vi "Create.vi"(7 "Registry Name":string, 8 "error in (no error)":errorcluster) -> (0 "error out":errorcluster, 3 "Process Collector out":refnum<class "Process Collector.lvclass">)   [LabVIEW 2020, in "Collector.lvlib" / "Process Collector.lvclass"]
uses:
  Process Collector.lvclass
  C:/Github-locals/PromVIEW/src/collector/collectable/Collectable.lvclass
  Process Collector.lvclass/Process Collector.ctl
  <vilib>/regexp/Match Regular Expression.xnode
  registry/session/Registry Session.lvclass
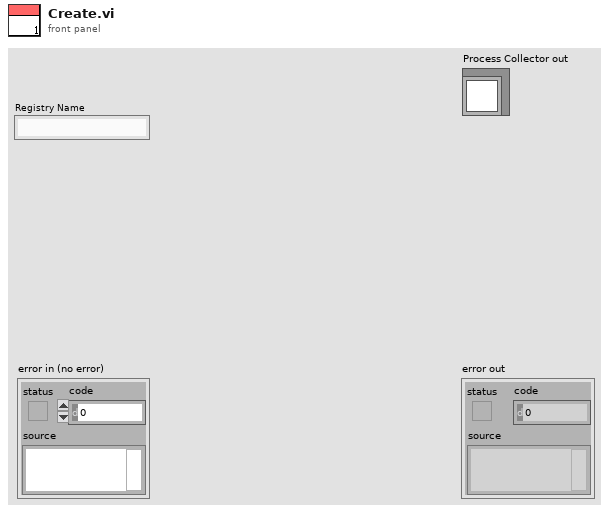
[diagram p1: front panel]
types:
  T1 = typedef "Registry.lvlib/Registry Session.lvclass/Session Handle.ctl" = refnum<data-value>
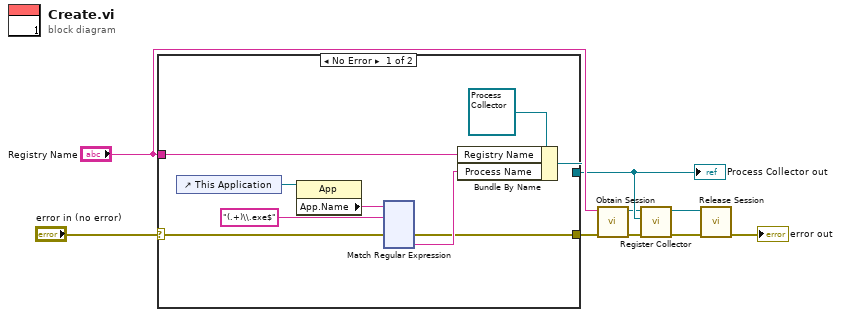
[diagram p0: block diagram]
diagram:
  n1 = case shown="No Error" "error in (no error)" {
    selector: "error in (no error)" -> [w13 w135]
    tunnel: [w12 w135] -> w1
    tunnel: [w18 _] -> w7
    tunnel: "Registry Name" -> [w10 _]
    frame No Error {
      n2 = control-ref of="This Application"() -> (w17:refnum<vi>)
      n3 = property class="App"(reference=w17) -> ("App.Name"=w16:string)  [unwired: 1 in, 2 out]
      n4 = xnode "Match Regular Expression"("input string"=w16, "regular expression"="(.+)\\.exe$", "error in"=w13) -> ("error out"=w12:errorcluster, "submatch 1"=w14:string)  [unwired: 3 in, 4 out]
      n5 = Bundle By Name(cluster=refnum<class "Process Collector.lvclass"> refnum ("Process Collector in"), "Registry Name"=w10, "Process Name"=w14) -> (w18:refnum<class "Process Collector.lvclass">)
    }
    frame Error {
    }
  }
  "Process Collector out" <- w7
  n6 = call "Obtain Session.vi"("error in (no error)"=w1, "Session  Name ()"="Registry Name") -> ("error out"=w5:errorcluster, "Session Handle"=w6:T1)  [unwired: 8 in]
  n7 = call "Register Collector.vi"("error in (no error)"=w5, "Collector"=w7, "Session Handle in"=w6) -> ("error out"=w3:errorcluster, "Session Handle out"=w4:T1)  [unwired: 7 in]
  n8 = call "Release Session.vi"("error in (no error)"=w3, "Session Handle"=w4) -> ("error out"=→"error out":errorcluster)  [unwired: 9 in]
